vi "read-sort-data.vi"(7 "all-data in":T1 {"dP3"."Temp (degC)" format="%.2f"; "dP3"."dP (mBar)" format="%.2f"; "dP2"."Temp (degC)" format="%.2f"; "dP2"."dP (mBar)" format="%.2f"; "dP1"."Temp (degC)" format="%.2f"; "dP1"."dP (mBar)" format="%.2f"; "CD4"."CO2 (ppm)" format="%.2f"; "CD3"."CO2 (ppm)" format="%.2f"; "RHT4"."Humidity (%)" format="%.2f"; "RHT4"."Temp (degC)" format="%.2f"; "RHT5"."Humidity (%)" format="%.2f"; "RHT5"."Temp (degC)" format="%.2f"; "CD2"."Humidity (%)" format="%.2f"; "CD2"."Temp (degC)" format="%.2f"; "CD2"."CO2 (ppm)" format="%.2f"; "RHT3"."Humidity (%)" format="%.2f"; "RHT3"."Temp (degC)" format="%.2f"; "CD6"."CO2 (ppm)" format="%.2f"; "RHT6"."Humidity (%)" format="%.2f"; "RHT6"."Temp (degC)" format="%.2f"; "CD5"."CO2 (ppm)" format="%.2f"; "CD1"."Humidity (%)" format="%.2f"; "CD1"."Temp (degC)" format="%.2f"; "CD1"."CO2 (ppm)" format="%.2f"}, 8 "error in (no error)":errorcluster, 11 "VISA Refnum in":refnum<visa-resource-name>) -> (0 "error out":errorcluster, 1 "timestamp":i32, 2 "all-data out":T1 {"dP3"."Temp (degC)" format="%.2f"; "dP3"."dP (mBar)" format="%.2f"; "dP2"."Temp (degC)" format="%.2f"; "dP2"."dP (mBar)" format="%.2f"; "dP1"."Temp (degC)" format="%.2f"; "dP1"."dP (mBar)" format="%.2f"; "CD4"."CO2 (ppm)" format="%.2f"; "CD3"."CO2 (ppm)" format="%.2f"; "RHT4"."Humidity (%)" format="%.2f"; "RHT4"."Temp (degC)" format="%.2f"; "RHT5"."Humidity (%)" format="%.2f"; "RHT5"."Temp (degC)" format="%.2f"; "CD2"."Humidity (%)" format="%.2f"; "CD2"."Temp (degC)" format="%.2f"; "CD2"."CO2 (ppm)" format="%.2f"; "RHT3"."Humidity (%)" format="%.2f"; "RHT3"."Temp (degC)" format="%.2f"; "CD6"."CO2 (ppm)" format="%.2f"; "RHT6"."Humidity (%)" format="%.2f"; "RHT6"."Temp (degC)" format="%.2f"; "CD5"."CO2 (ppm)" format="%.2f"; "CD1"."Humidity (%)" format="%.2f"; "CD1"."Temp (degC)" format="%.2f"; "CD1"."CO2 (ppm)" format="%.2f"}, 3 "VISA Refnum out":refnum<visa-resource-name>, 4 "read buffer":string)   [LabVIEW 2021]
uses:
  all-sensor-data.ctl
  SCD41.ctl
  STC31.ctl
  SHT41.ctl
  SDP810.ctl
panel:
  out "read buffer out":string
  out "data string array":string[](array[string])
  out "Bytes Returned":u32
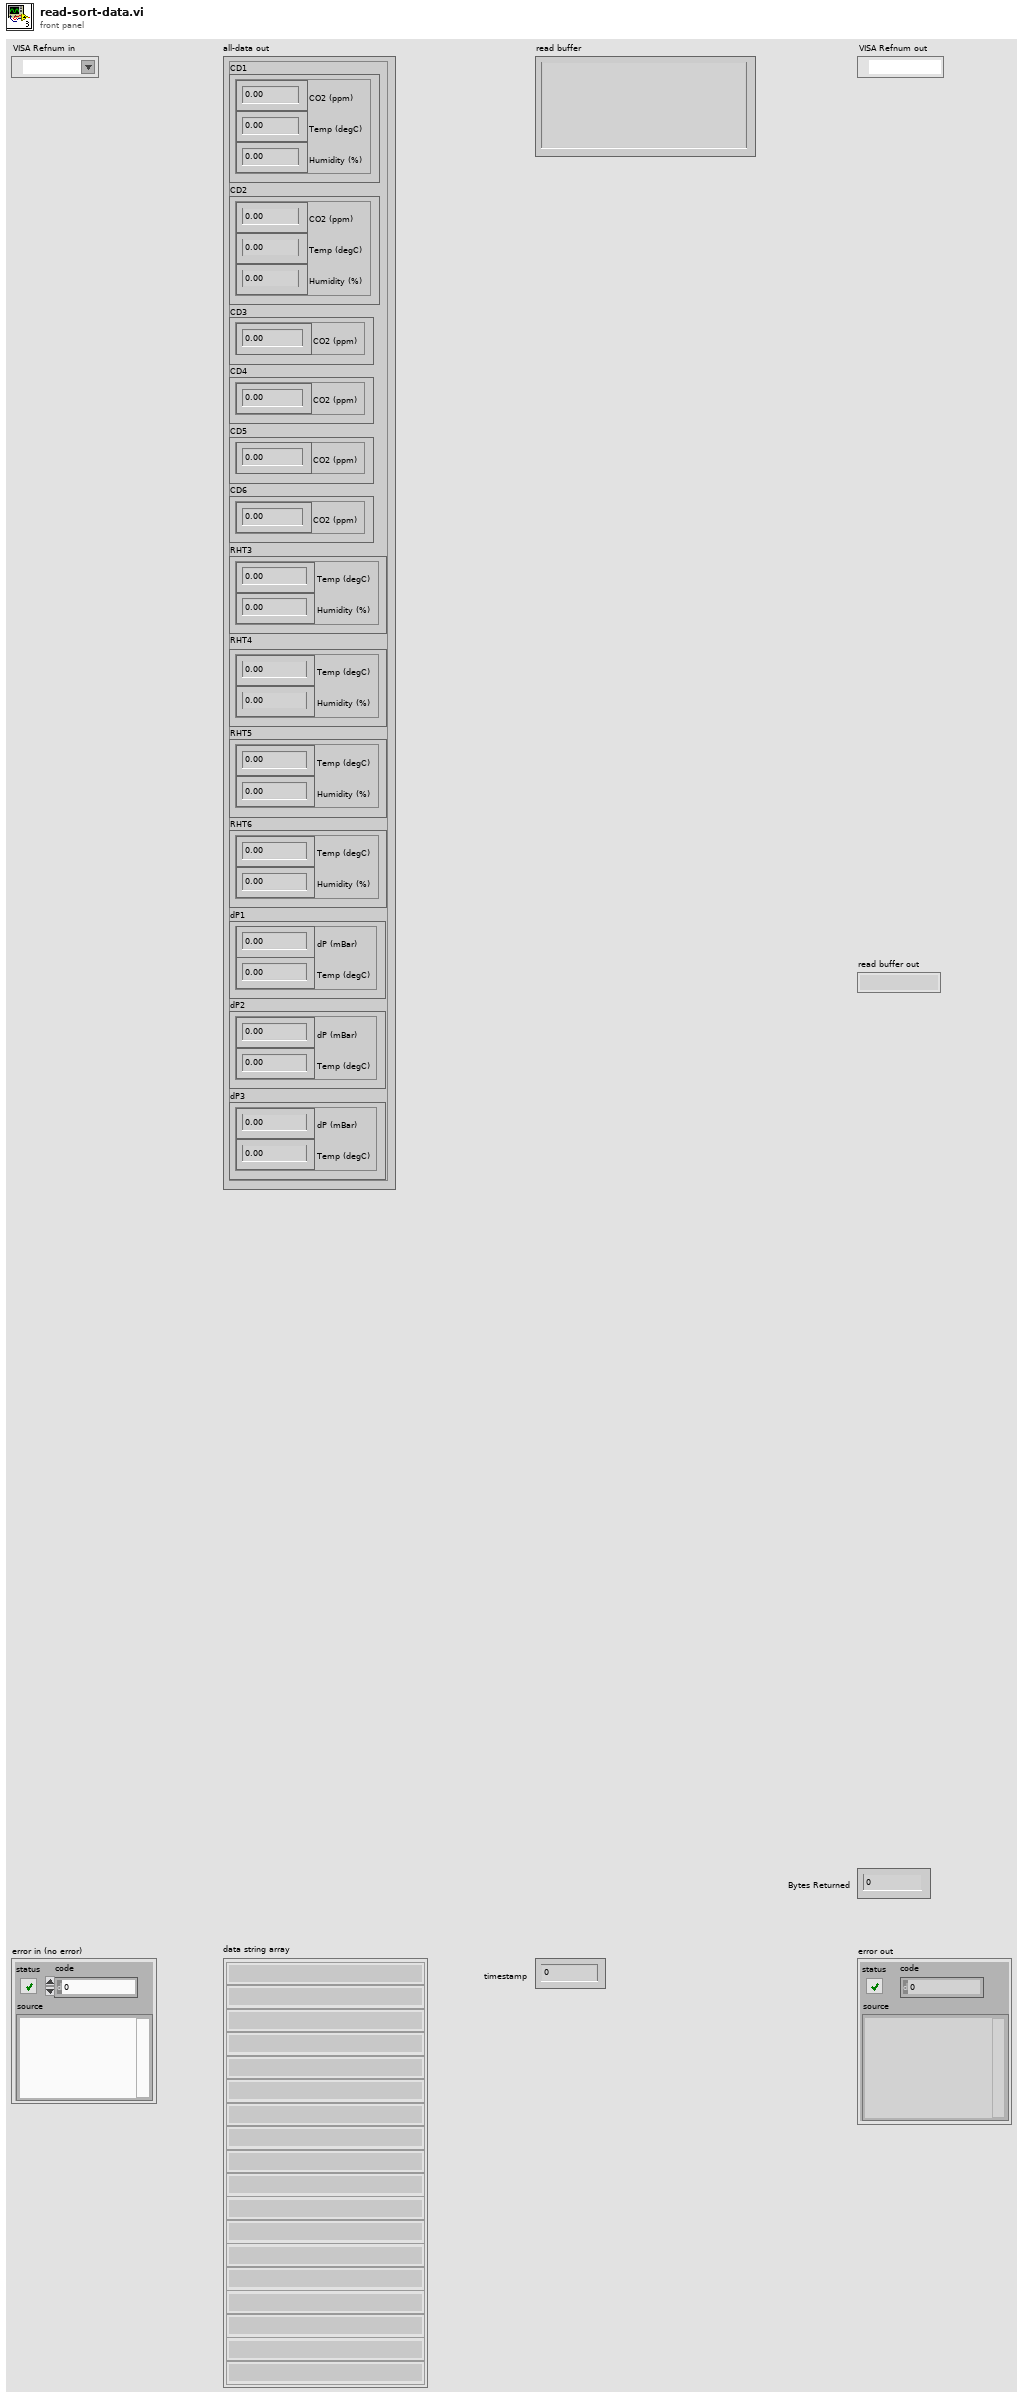
[diagram p1: front panel]
types:
  T1 = typedef "all-sensor-data.ctl" = cluster{"CD1":T2, "CD2":T2, "CD3":T3, "CD4":T3, "CD5":T3, "CD6":T3, "RHT3":T4, "RHT4":T4, "RHT5":T4, "RHT6":T4, "dP1":T5, "dP2":T5, "dP3":T5}
  T2 = typedef "SCD41.ctl" = cluster{"CO2 (ppm)":dbl, "Temp (degC)":dbl, "Humidity (%)":dbl}
  T3 = typedef "STC31.ctl" = cluster{"CO2 (ppm)":dbl}
  T4 = typedef "SHT41.ctl" = cluster{"Temp (degC)":dbl, "Humidity (%)":dbl}
  T5 = typedef "SDP810.ctl" = cluster{"dP (mBar)":dbl, "Temp (degC)":dbl}
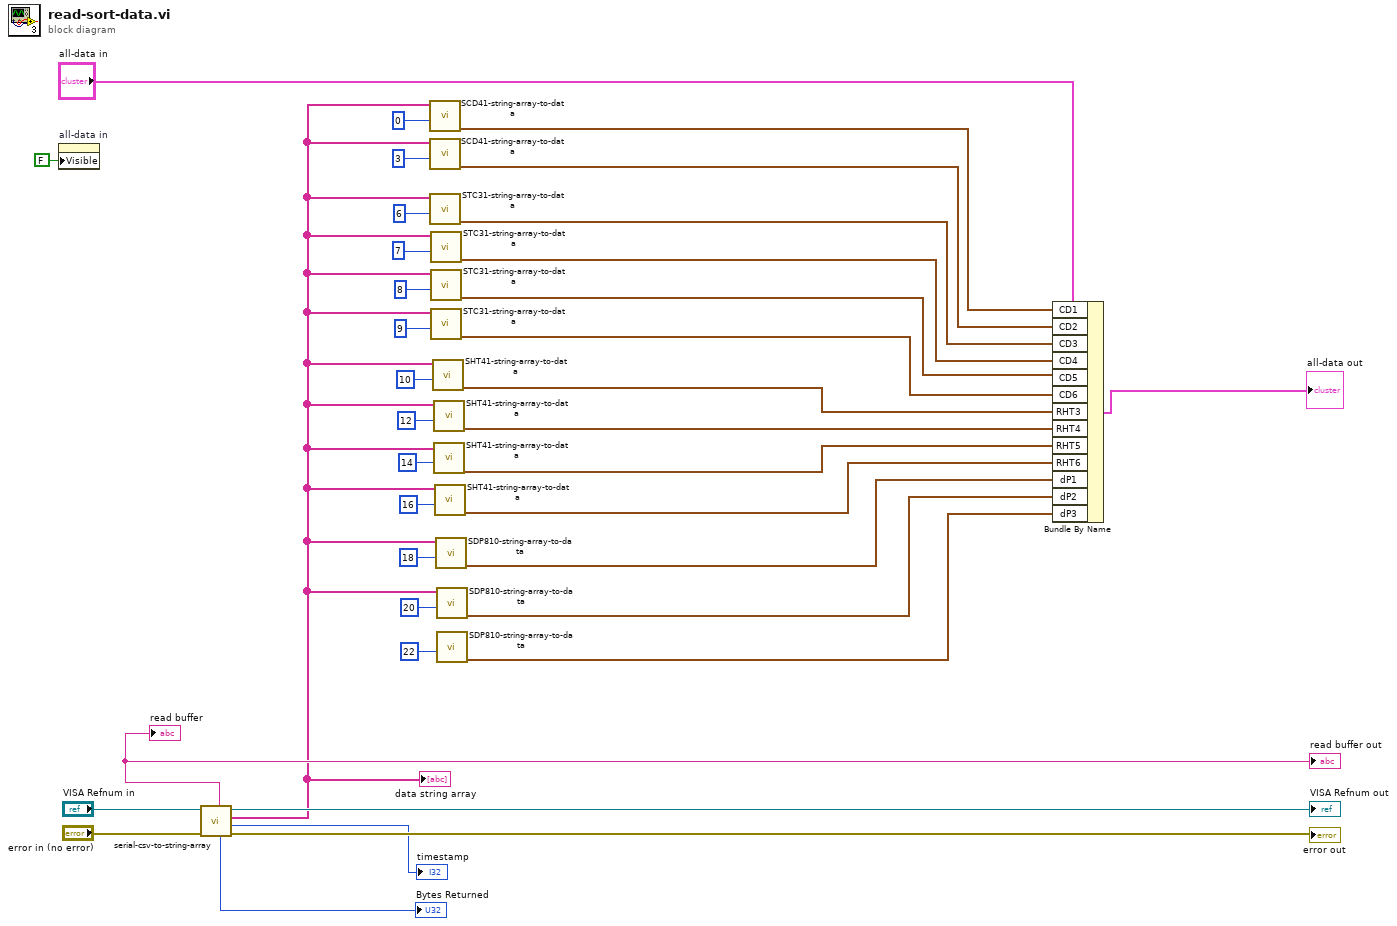
[diagram p0: block diagram]
diagram:
  n1 = property on="all-data in" class="Clust (strict)"("Visible"=FALSE) -> ()  [unwired: 2 in, 2 out]
  n2 = call "serial-csv-to-string-array.vi"("error in (no error)"="error in (no error)", "VISA Refnum in"="VISA Refnum in") -> ("error out"=→"error out":errorcluster, "timestamp"=→"timestamp":i32, "data string array"=w3:string[], "VISA Refnum out"=→"VISA Refnum out":refnum<visa-resource-name>, "Bytes Returned"=→"Bytes Returned":u32, "read buffer"=→"read buffer" →"read buffer out":string)  [unwired: 4 in]
  "data string array" <- w3
  n3 = call "SCD41-string-array-to-data.vi"("Starting Index"=0, "Data In (string array)"=w3) -> ("SCD41: data output"=w23:T2)  [unwired: 6 in, 3 out]
  n4 = call "SCD41-string-array-to-data.vi"("Starting Index"=3, "Data In (string array)"=w3) -> ("SCD41: data output"=w24:T2)  [unwired: 6 in, 3 out]
  n5 = call "STC31-string-array-to-data.vi"("Starting Index"=6 ("index"), "Data In (string array)"=w3) -> ("STC31: data output"=w25:T3)  [unwired: 7 in, 2 out]
  n6 = call "STC31-string-array-to-data.vi"("Starting Index"=7, "Data In (string array)"=w3) -> ("STC31: data output"=w26:T3)  [unwired: 7 in, 2 out]
  n7 = call "STC31-string-array-to-data.vi"("Starting Index"=8, "Data In (string array)"=w3) -> ("STC31: data output"=w8:T3)  [unwired: 7 in, 2 out]
  n8 = call "STC31-string-array-to-data.vi"("Starting Index"=9, "Data In (string array)"=w3) -> ("STC31: data output"=w27:T3)  [unwired: 7 in, 2 out]
  n9 = call "SHT41-string-array-to-data.vi"("Starting Index"=10, "Data In (string array)"=w3) -> ("SHT41: data output"=w28:T4)  [unwired: 7 in, 2 out]
  n10 = call "SHT41-string-array-to-data.vi"("Starting Index"=12, "Data In (string array)"=w3) -> ("SHT41: data output"=w29:T4)  [unwired: 7 in, 2 out]
  n11 = call "SHT41-string-array-to-data.vi"("Starting Index"=14, "Data In (string array)"=w3) -> ("SHT41: data output"=w30:T4)  [unwired: 7 in, 2 out]
  n12 = call "SHT41-string-array-to-data.vi"("Starting Index"=16, "Data In (string array)"=w3) -> ("SHT41: data output"=w31:T4)  [unwired: 7 in, 2 out]
  n13 = call "SDP810-string-array-to-data.vi"("Starting Index"=18, "Data In (string array)"=w3) -> ("SDP810: data output"=w6:T4)  [unwired: 7 in, 2 out]
  n14 = call "SDP810-string-array-to-data.vi"("Starting Index"=20, "Data In (string array)"=w3) -> ("SDP810: data output"=w5:T4)  [unwired: 7 in, 2 out]
  n15 = call "SDP810-string-array-to-data.vi"("Starting Index"=22) -> ("SDP810: data output"=w1:T4)  [unwired: 8 in, 2 out]
  n16 = Bundle By Name(cluster="all-data in", "CD1"=w23, "CD2"=w24, "CD3"=w25, "CD4"=w26, "CD5"=w8, "CD6"=w27, "RHT3"=w28, "RHT4"=w29, "RHT5"=w30, "RHT6"=w31, "dP1"=w6, "dP2"=w5, "dP3"=w1) -> (→"all-data out":T1)
